vi "Scale Points.vi"(8 "Z Scale":dbl, 9 "Y Scale":dbl, 10 "X Scale":dbl, 11 "In Points":i32[][](array[numeric])) -> (3 "Scaled Points":dbl[][](array[numeric]))   [LabVIEW 2013]
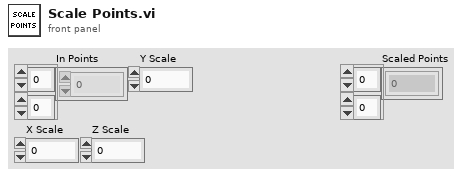
[diagram p1: front panel]
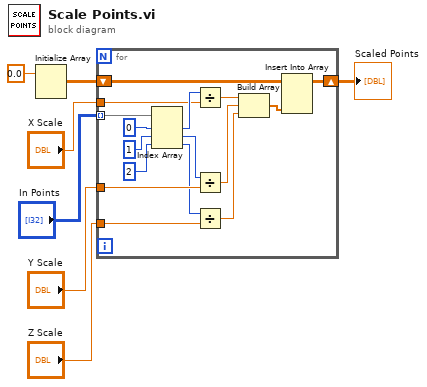
[diagram p0: block diagram]
diagram:
  n1 = Initialize Array(0.0 ("element")) -> (w6:dbl[][])  [unwired: 2 in]
  n2 = for {
    tunnel: "In Points" -> [w23] mode=indexing
    tunnel: "Y Scale" -> [w18]
    tunnel: "X Scale" -> [w17]
    shift-right: [w11] -> w5
    shift-left: w6 -> [w13]
    tunnel: "Z Scale" -> [w8]
    n3 = Index Array(array=w23, index #1=0 ("index"), index #2=1 ("index"), index #3=2 ("index")) -> (element #1=w20:i32, element #2=w19:i32, element #3=w9:i32)
    n4 = Divide(x=w20, y=w17) -> (x/y=w15:dbl)
    n5 = Divide(x=w19, y=w18) -> (x/y=w14:dbl)
    n6 = Divide(x=w9, y=w8) -> (x/y=w10:dbl)
    n7 = Build Array(w15, w14, w10) -> (w12:dbl[])
    n8 = Insert Into Array(array=w13, new element=w12) -> (w11:dbl[][])  [unwired: 2 in]
  }
  "Scaled Points" <- w5
